vi "pallet DB 2.vi"(0 "pallet_num":i32, 2 "info array":dbl[][](array[numeric]), 6 "set data":bool, 9 "error in":errorcluster) -> (27 "error out":errorcluster)   [LabVIEW 2019]
uses:
  <vilib>/addons/database/Auxilliary.llb/DB Tools Format Datetime String (Time Stamp).vi
  <vilib>/addons/database/NI_Database_API.lvlib
  database.lvlib
panel:
  # "Database table"
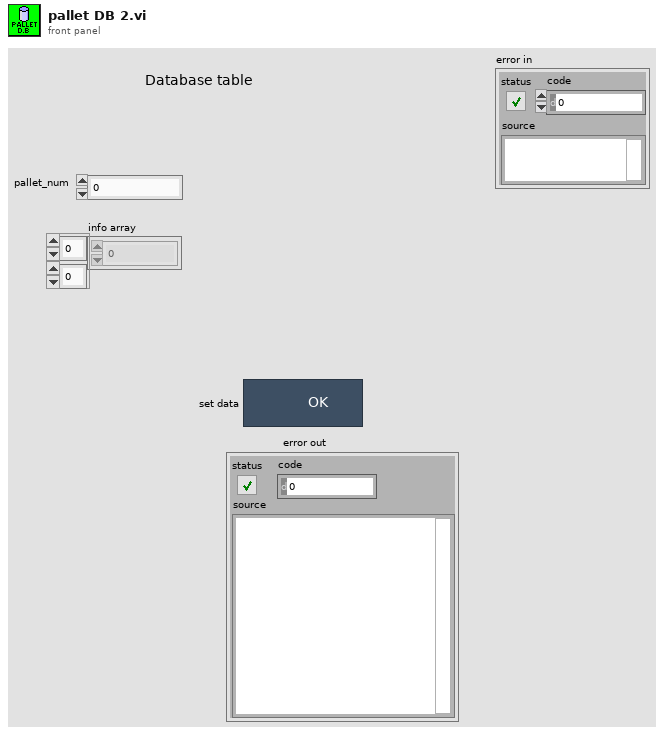
[diagram p1: front panel]
types:
  T1 = cluster{"plt number dis":i16, "Table Name":string, "Database Name":string, "DB days to save":i16, "IP #":string, "Img Path":path, "Port":u16, "time out":u16, "madule path":path, "IP # speed":string, "counting device":enum16{"Sensors", "Line Speed", "Sensors&Speed"}}
  T2 = cluster{string, "date/time string":string, string, "f":string, string, string, string, string, string, string, string, string, string, string, string}
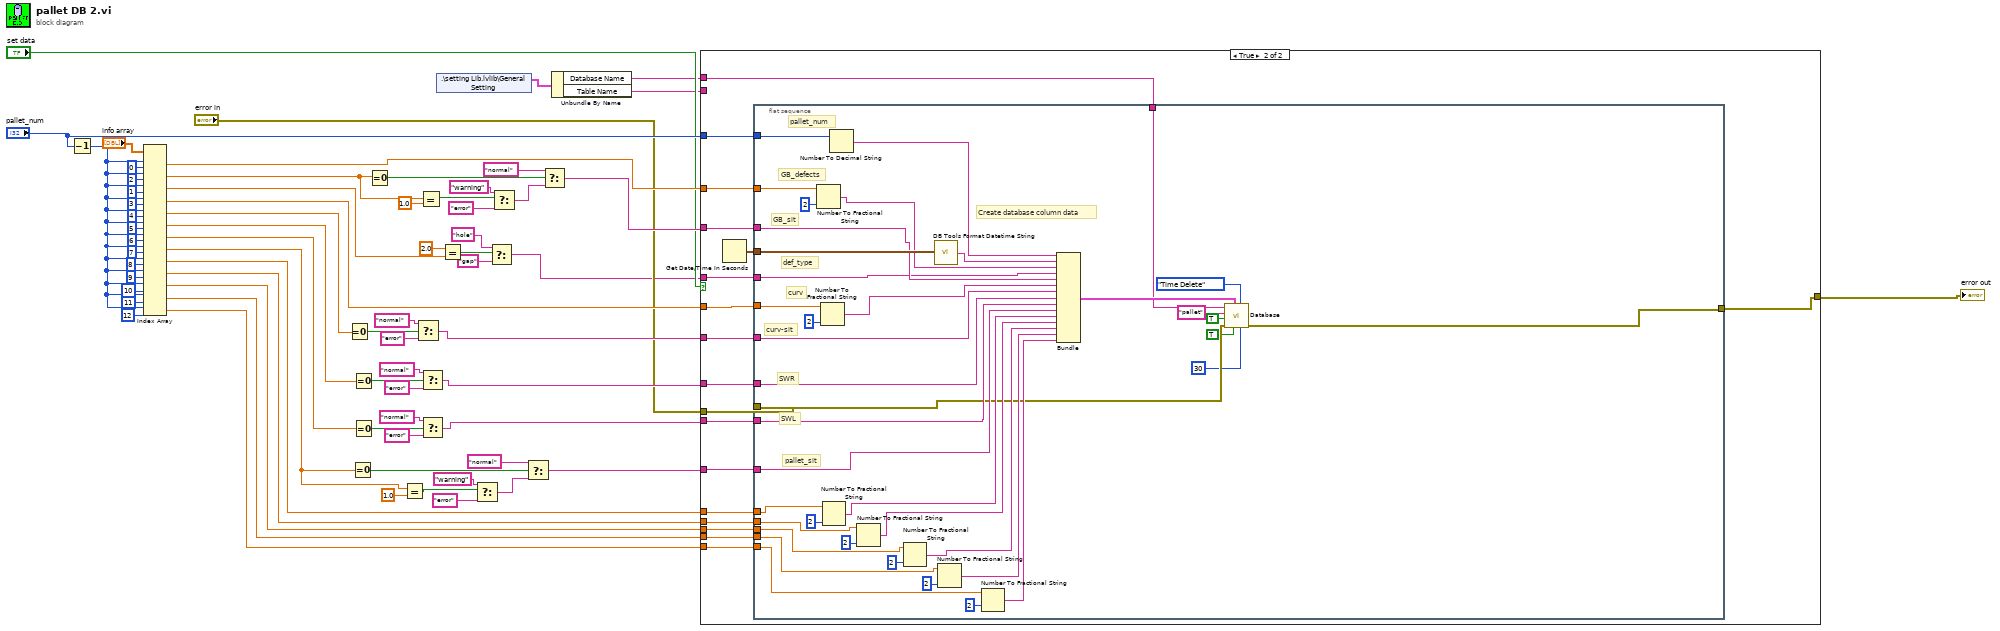
[diagram p0: block diagram]
diagram:
  n1 = Decrement(x="pallet_num") -> (x-1=w23:i32)
  n2 = Index Array(array="info array", index (row) #1=w23, index (col) #1=0 ("disabled index (col)"), index (row) #2=w23, index (col) #2=2 ("disabled index (col)"), index (row) #3=w23, index (col) #3=1 ("disabled index (col)"), index (row) #4=w23, index (col) #4=3 ("disabled index (col)"), index (row) #5=w23, index (col) #5=4 ("disabled index (col)"), index (row) #6=w23, index (col) #6=5 ("disabled index (col)"), index (row) #7=w23, index (col) #7=6 ("disabled index (col)"), index (row) #8=w23, index (col) #8=7 ("disabled index (col)"), index (row) #9=w23, index (col) #9=8 ("disabled index (col)"), index (row) #10=w23, index (col) #10=9 ("disabled index (col)"), index (row) #11=w23, index (col) #11=10 ("disabled index (col)"), index (row) #12=w23, index (col) #12=11 ("disabled index (col)"), index (row) #13=w23, index (col) #13=12 ("disabled index (col)")) -> (element #1=w59:dbl, element #2=w54:dbl, element #3=w9:dbl, element #4=w49:dbl, element #5=w48:dbl, element #6=w37:dbl, element #7=w36:dbl, element #8=w25:dbl, element #9=w17:dbl, element #10=w16:dbl, element #11=w15:dbl, element #12=w14:dbl, element #13=w13:dbl)
  n3 = Equal To 0?(x=w48) -> (x = 0?=w47:bool)
  n4 = Equal To 0?(x=w25) -> (x = 0?=w26:bool)
  n5 = Equal To 0?(x=w37) -> (x = 0?=w41:bool)
  n6 = Equal To 0?(x=w36) -> (x = 0?=w40:bool)
  n7 = Equal To 0?(x=w54) -> (x = 0?=w58:bool)
  n8 = Equal?(x=w25, y=1.0) -> (x = y?=w31:bool)
  n9 = Select(t="normal", s=w47, f="error") -> (s? t:f=w44:string)
  n10 = Equal?(x=w54, y=1.0) -> (x = y?=w52:bool)
  n11 = Select(t="normal", s=w41, f="error") -> (s? t:f=w35:string)
  n12 = Select(t="normal", s=w40, f="error") -> (s? t:f=w34:string)
  n13 = shared-variable ".\\setting Lib.lvlib\\General Setting"() -> (w3:T1)  [unwired: 1 in, 1 out]
  n14 = Equal?(x=2.0, y=w9) -> (x = y?=w8:bool)
  n15 = Select(t="warning", s=w31, f="error") -> (s? t:f=w32:string)
  n16 = Select(t="hole", s=w8, f="gap") -> (s? t:f=w5:string)
  n17 = Select(t="warning", s=w52, f="error") -> (s? t:f=w51:string)
  n18 = Select(t="normal", s=w26, f=w32) -> (s? t:f=w24:string)
  n19 = Select(t="normal", s=w58, f=w51) -> (s? t:f=w50:string)
  n20 = Unbundle By Name(w3) -> ("Database Name"=w2:string, "Table Name"=w1:string)
  n21 = case shown="True" "set data" {
    tunnel: "error in" -> [w69 w87]
    tunnel: [w69 w85] -> w10
    tunnel: "pallet_num" -> [_ w84]
    tunnel: w59 -> [_ w83]
    tunnel: w50 -> [_ w82]
    tunnel: w49 -> [_ w81]
    tunnel: w44 -> [_ w80]
    tunnel: w35 -> [_ w79]
    tunnel: w34 -> [_ w78]
    tunnel: w24 -> [_ w77]
    tunnel: w17 -> [_ w76]
    tunnel: w16 -> [_ w75]
    tunnel: w15 -> [_ w74]
    tunnel: w14 -> [_ w73]
    tunnel: w13 -> [_ w72]
    tunnel: w5 -> [_ w71]
    tunnel: w2 -> [_ w70]
    tunnel: w1 -> [_ _]
    frame False {
    }
    frame True {
      n22 = Get Date/Time In Seconds() -> (seconds since 1Jan1904=w86:timestamp)
      n23 = flat-sequence {
        tunnel: [w93] -> w85
        tunnel: w72 -> [w108]
        tunnel: w73 -> [w109]
        tunnel: w74 -> [w110]
        tunnel: w75 -> [w111]
        tunnel: w76 -> [w112]
        tunnel: w77 -> [w114]
        tunnel: w78 -> [w115]
        tunnel: w79 -> [w116]
        tunnel: w80 -> [w117]
        tunnel: w81 -> [w118]
        tunnel: w82 -> [w113]
        tunnel: w83 -> [w119]
        tunnel: w84 -> [w120]
        tunnel: w86 -> [w126]
        tunnel: w87 -> [w95]
        tunnel: w71 -> [w97]
        tunnel: w70 -> [w94]
        frame #0 {
          # "pallet_sit"
          # "SWL"
          # "SWR"
          # "curv-sit"
          # "curv"
          # "def_type"
          # "GB_sit"
          # "GB_defects"
          # "pallet_num"
          # "Create database column data"
          n24 = Number To Fractional String(number=w119, precision (6)=i16 2) -> (F-format string=w124:string)  [unwired: 2 in]
          n25 = Number To Fractional String(number=w118, precision (6)=i16 2) -> (F-format string=w121:string)  [unwired: 2 in]
          n26 = Number To Fractional String(number=w112, precision (6)=i16 2) -> (F-format string=w102:string)  [unwired: 2 in]
          n27 = Number To Decimal String(number=w120) -> (decimal integer string=w125:string)  [unwired: 1 in]
          n28 = Number To Fractional String(number=w111, precision (6)=i16 2) -> (F-format string=w101:string)  [unwired: 2 in]
          n29 = Number To Fractional String(number=w110, precision (6)=i16 2) -> (F-format string=w100:string)  [unwired: 2 in]
          n30 = call-poly <vilib>:"DB Tools Format Datetime String.vi"("time stamp"=w126) -> ("date/time string"=w127:string)
          n31 = Number To Fractional String(number=w109, precision (6)=i16 2) -> (F-format string=w99:string)  [unwired: 2 in]
          n32 = Number To Fractional String(number=w108, precision (6)=i16 2) -> (F-format string=w98:string)  [unwired: 2 in]
          n33 = Bundle(w125, "date/time string"=w127, w124, "f"=w97, w113, w121, w117, w116, w115, w114, w102, w101, w100, w99, w98) -> (w96:T2)  [unwired: 1 in]
          n34 = call "Database.vi"("Maximum Row"=30, "Enum"=enum16{"ID Delete", "Time Delete"}."Time Delete", "Delete row?"=TRUE, "Data"=w96, "Error in"=w95, "Auto Increment ID?"=TRUE, "Table"="pallet", "Connection"=w94) -> ("Error out"=w93:errorcluster)  [unwired: 3 in]
        }
      }
    }
  }
  "error out" <- w10
